vi "LBCB Cartesian Data.vi"() -> ()   [LabVIEW 2009]
uses:
  lib/Launcher/Launcher Actions.ctl
  lib/Launcher/NoPanelAppTypes.ctl
  lib/Data Access Objects/Metadata/DAO Actions.ctl
  lib/Data Access Objects/Application/Number Of LBCBs.ctl
  lib/Data Access Objects/Metadata/Persistant DAO Actions.ctl
panel:
  in  "Force Offset Tag":u16(ring)
  in  "Cartesian Type":bool caption="Coord"
  in  "Label1 3":string="Combined"
  in  "Label1 2":string="LBCB 2"
  in  "Label1":string="LBCB 1"
  out "Combined Data":dbl[][](array[numeric]) caption="LBCB 2 Data"
  out "DOF Labels3":string[](array[string])=["Dx", "Dy", "Dz", "Rx", "Ry", "Rz"]
  out "LBCB 1 Data":dbl[][](array[numeric])
  out "LBCB 2 Data":dbl[][](array[numeric])
  out "DOF Labels 2":string[](array[string])=["Dx", "Dy", "Dz", "Rx", "Ry", "Rz"]
  out "DOF Labels":string[](array[string])=["Dx", "Dy", "Dz", "Rx", "Ry", "Rz"]
  in  "Ok":bool
  # "Forces"
  # "Displacements"
  # "Commands"
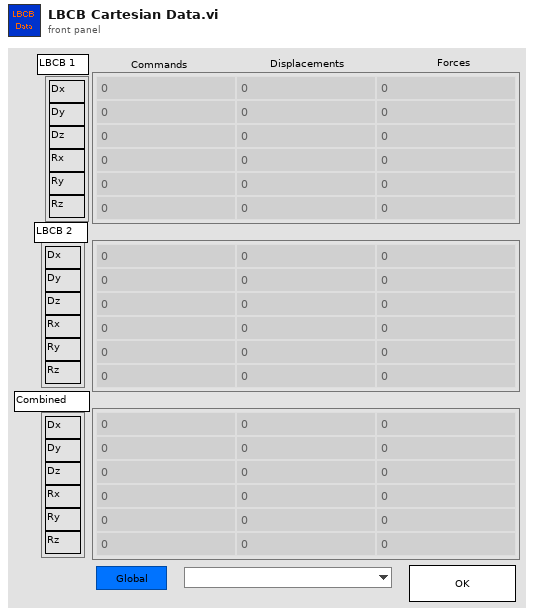
[diagram p1: front panel]
types:
  T1 = typedef "NoPanelAppTypes.ctl" = enum16{"NTCP Socket", "Data Archiving", "DAQ Link", "Control Loops", "Cmd Disp Diffs", "LBCB Cart Data", "Limits", "Mixed Mode Widget", "Offsets"}
  T2 = typedef "Launcher Actions.ctl" = enum16{"Launch", "Stop All", "Stop", "Kill", "Running?", "Init"}
  T3 = typedef "DAO Actions.ctl" = enum16{"Init", "Get", "Set"}
  T4 = typedef "Number Of LBCBs.ctl" = enum16{"1", "2"}
  T5 = typedef "Persistant DAO Actions.ctl" = enum16{"Init", "Get", "Set", "Load", "Save"}
  T6 = typedef "Dataset Source.ctl" = enum16{"LBCB 1", "LBCB 2", "Combined", "External Sensors"}
  T7 = typedef "Dataset Transaction Id.ctl" = cluster{"Dataset Source":T6, "Dataset Type":T8, "Hold":T9, "Volts":T9, "Tag":string}
  T8 = typedef "Dataset Type.ctl" = enum16{"LVDT", "Load Cell", "Actuator Command", "Servo Error", "Displacement Command", "Displacement", "Force"}
  T9 = typedef "Yes No Button.ctl" = bool
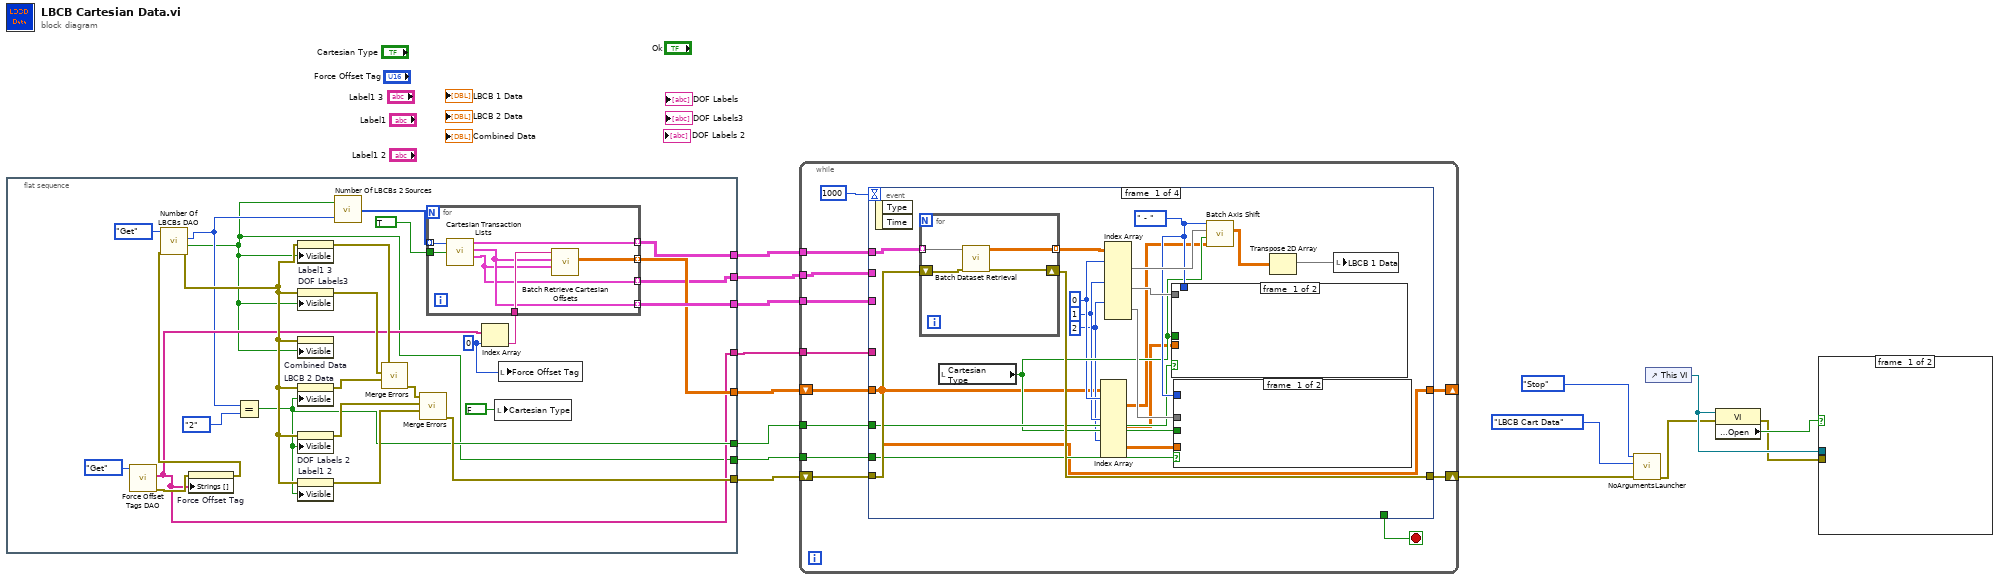
[diagram p0: block diagram]
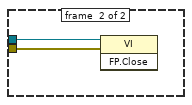
[diagram p2: hidden frame]
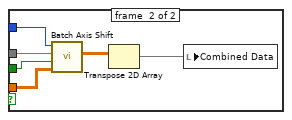
[diagram p3: hidden frame]
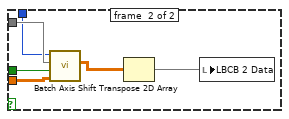
[diagram p4: hidden frame]
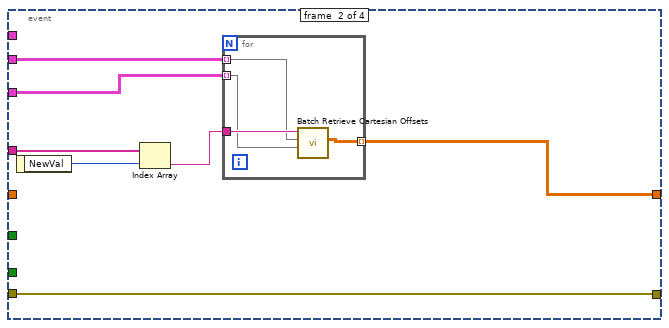
[diagram p5: hidden frame]
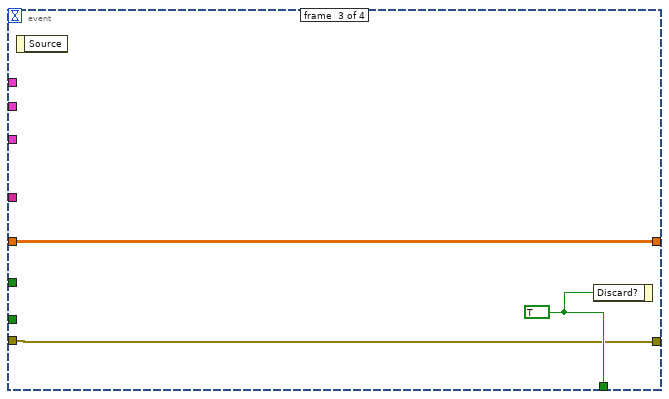
[diagram p6: hidden frame]
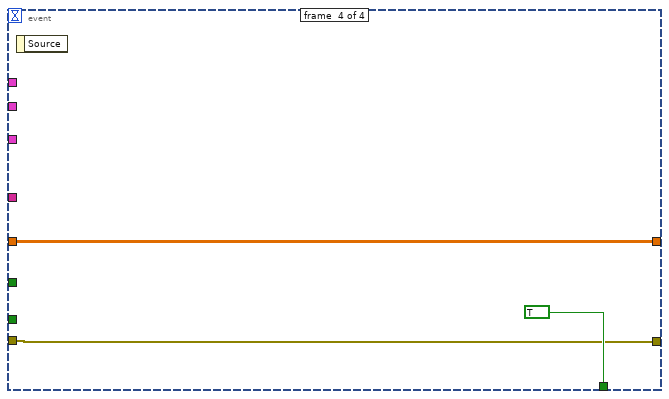
[diagram p7: hidden frame]
diagram:
  n1 = flat-sequence {
    tunnel: [w41] -> w12
    tunnel: [w25] -> w11
    tunnel: [w24] -> w10
    tunnel: [w18] -> w9
    tunnel: [w23] -> w8
    tunnel: [w22] -> w7
    tunnel: [w21] -> w6
    tunnel: [w20] -> w5
    frame #0 {
      w28 = 0 ("index")
      n2 = call "Force Offset Tags DAO.vi"("DAO Actions"=DAO_Actions."Get") -> ("error out"=w30:errorcluster, "Force Tags"=w20:string[])  [unwired: 9 in]
      n3 = property on="Force Offset Tag" class="Ring (strict)"(error in=w30, "Strings []"=w20) -> (error out=w29:errorcluster)  [unwired: 1 in, 1 out]
      n4 = call "Number Of LBCBs DAO.vi"("error in (no error)"=w29, "Actions"=Persistant_DAO_Actions."Get") -> ("error out"=w38:errorcluster, "Rigid Connection Out"=w18:bool, "Number of\nLBCBs Out"=w19:T4)  [unwired: 6 in, 1 out]
      n5 = Equal?(x=w19, y=Number_Of_LBCBs."2") -> (x = y?=w23:bool)
      n6 = property on="Label1 3" class="Str"(error in=w38, "Visible"=w18) -> (error out=w37:errorcluster)  [unwired: 1 in, 1 out]
      n7 = property on="DOF Labels3" class="Arr (strict)"(error in=w38, "Visible"=w18) -> (error out=w36:errorcluster)  [unwired: 1 in, 1 out]
      n8 = property on="Combined Data" class="Arr (strict)"(error in=w38, "Visible"=w18) -> ()  [unwired: 1 in, 2 out]
      n9 = property on="LBCB 2 Data" class="Arr (strict)"(error in=w38, "Visible"=w23) -> (error out=w35:errorcluster)  [unwired: 1 in, 1 out]
      n10 = property on="DOF Labels 2" class="Arr (strict)"(error in=w38, "Visible"=w23) -> (error out=w33:errorcluster)  [unwired: 1 in, 1 out]
      n11 = property on="Label1 2" class="Str"(error in=w38, "Visible"=w23) -> (error out=w32:errorcluster)  [unwired: 1 in, 1 out]
      n12 = call "Number Of LBCBs 2 Sources.vi"("Number of LBCBs"=w19, "Combined LBCBs"=w18) -> ("Sources"=w17:T6[])
      n13 = call <vilib>:"Merge Errors.vi"("error in 3 (no error)"=w35, "error in 2 (no error)"=w36, "error in 1 (no error)"=w37) -> ("error out"=w34:errorcluster)  [unwired: 4 in]
      n14 = call <vilib>:"Merge Errors.vi"("error in 3 (no error)"=w32, "error in 2 (no error)"=w33, "error in 1 (no error)"=w34) -> ("error out"=w41:errorcluster)  [unwired: 4 in]
      n15 = Index Array(array=w20, index=w28) -> (element=w26:string)
      n16 = for {
        tunnel: w26 -> [w48]
        tunnel: [w47] -> w25 mode=indexing
        tunnel: [w46] -> w24 mode=indexing
        tunnel: [w45] -> w22 mode=indexing
        tunnel: [w44] -> w21 mode=indexing
        tunnel: w17 -> [w43] mode=indexing
        tunnel: TRUE ("Include Command") -> [w42]
        n17 = call "Cartesian Transaction Lists.vi"("Source"=w43, "Include Command"=w42) -> ("Cartesian Data"=w47:T7[], "Displacement Offsets"=w46:T7[], "Force Offsets"=w44:T7[])  [unwired: 1 in, 1 out]
        n18 = call "Batch Retrieve Cartesian Offsets.vi"("Force Offsets"=w44, "Displacement Offsets"=w46, "Force Tag"=w48) -> ("Offsets"=w45:dbl[][])  [unwired: 5 in, 1 out]
      }
      n19 = local write "Cartesian Type"(FALSE ("Cartesian Type")) -> ()
      n20 = local write "Force Offset Tag"(w28) -> ()
    }
  }
  n21 = while {
    shift-right: [w57] -> w13
    shift-left: w12 -> [w58]
    tunnel: w11 -> [w56]
    tunnel: w10 -> [w50]
    tunnel: w9 -> [w55]
    tunnel: w8 -> [w54]
    shift-right: [w49] -> _
    shift-left: w7 -> [w53]
    tunnel: w6 -> [w51]
    tunnel: w5 -> [w52]
    stop <- w59 stop-if-true
    n22 = event shown="[3] Application Instance Close;  Panel Close" {
      selector: _ -> [_ _ _ _]
      dyn-events: _ -> [_ _ _ _]
      timeout: 1000 -> [_ _ _ _]
      tunnel: [_ _ w110 TRUE] -> w59
      tunnel: w58 -> [w80 w97 w109 w112]
      tunnel: [w79 w97 w109 w112] -> w57
      tunnel: w56 -> [w76 _ _ _]
      tunnel: w55 -> [w71 _ _ _]
      tunnel: w54 -> [w69 _ _ _]
      tunnel: w53 -> [w61 _ w108 w111]
      tunnel: w52 -> [_ w103 _ _]
      tunnel: w51 -> [_ w100 _ _]
      tunnel: w50 -> [_ w99 _ _]
      tunnel: [w61 w98 w108 w111] -> w49
      event #0 {
        w70 = enum16{" +", " - "}." - " ("Direction")
        w65 = 2 ("index (row)")
        w66 = 1 ("index (row)")
        w67 = 0 ("index (row)")
        n23 = event-data() -> ()  [unwired: 3 out]
        n24 = for {
          tunnel: w76 -> [w96] mode=indexing
          shift-right: [w94] -> w79
          shift-left: w80 -> [w95]
          tunnel: [w93] -> w78 mode=indexing
          n25 = call "Batch Dataset Retrieval.vi"("error in"=w95, "Transactions"=w96) -> ("error out"=w94:errorcluster, "Data"=w93:dbl[][])  [unwired: 8 in]
        }
        n26 = local read "Cartesian Type"() -> (w68:bool)
        n27 = Index Array(array=w61, index (dim 0) #1=w67, index (dim 0) #2=w66, index (dim 0) #3=w65) -> (element #1=w64:dbl[][], element #2=w63:dbl[][], element #3=w62:dbl[][])  [unwired: 6 in]
        n28 = Index Array(array=w78, index (dim 0) #1=w67, index (dim 0) #2=w66, index (dim 0) #3=w65) -> (element #1=w75:dbl[][], element #2=w73:dbl[][], element #3=w72:dbl[][])  [unwired: 6 in]
        n29 = case shown="True" w69 {
          tunnel: w73 -> [_ w91]
          tunnel: w70 -> [_ w89]
          tunnel: w68 -> [_ w88]
          tunnel: w63 -> [_ w87]
          frame #0 {
          }
          frame #1 {
            n30 = call "Batch Axis Shift.vi"("Offsets In"=w87, "Coordinate Switch"=w88, "Data In"=w91, "Direction"=w89) -> ("Data Out"=w90:dbl[][])  [unwired: 7 in]
            n31 = Transpose 2D Array(2D array=w90) -> (transposed array=w92:dbl[][])
            n32 = local write "LBCB 2 Data"(w92) -> ()
          }
        }
        n33 = case shown="True" w71 {
          tunnel: w72 -> [_ w85]
          tunnel: w70 -> [_ w83]
          tunnel: w68 -> [_ w82]
          tunnel: w62 -> [_ w81]
          frame #0 {
          }
          frame #1 {
            n34 = call "Batch Axis Shift.vi"("Offsets In"=w81, "Coordinate Switch"=w82, "Data In"=w85, "Direction"=w83) -> ("Data Out"=w84:dbl[][])  [unwired: 7 in]
            n35 = Transpose 2D Array(2D array=w84) -> (transposed array=w86:dbl[][])
            n36 = local write "Combined Data"(w86) -> ()
          }
        }
        n37 = call "Batch Axis Shift.vi"("Offsets In"=w64, "Coordinate Switch"=w68, "Data In"=w75, "Direction"=w70) -> ("Data Out"=w74:dbl[][])  [unwired: 7 in]
        n38 = Transpose 2D Array(2D array=w74) -> (transposed array=w77:dbl[][])
        n39 = local write "LBCB 1 Data"(w77) -> ()
      }
      event #1 {
        n40 = event-data() -> ("NewVal"=w102:u16)  [unwired: 1 out]
        n41 = Index Array(array=w103, index=w102) -> (element=w101:string)
        n42 = for {
          tunnel: w101 -> [w107]
          tunnel: w100 -> [w106] mode=indexing
          tunnel: w99 -> [w105] mode=indexing
          tunnel: [w104] -> w98 mode=indexing
          n43 = call "Batch Retrieve Cartesian Offsets.vi"("Force Offsets"=w105, "Displacement Offsets"=w106, "Force Tag"=w107) -> ("Offsets"=w104:dbl[][])  [unwired: 5 in, 1 out]
        }
      }
      event #2 {
        w110 = TRUE
        n44 = event-data() -> ()  [unwired: 2 out]
        n45 = event-data("Discard?"=w110) -> ()  [unwired: 1 in, 1 out]
      }
      event #3 {
        n46 = event-data() -> ()  [unwired: 2 out]
      }
    }
  }
  n47 = call "NoArgumentsLauncher.vi"("error in (no error)"=w13, "Application"=NoPanelAppTypes."LBCB Cart Data", "Application Launcher Actions"=Launcher_Actions."Stop") -> ("error out"=w2:errorcluster)  [unwired: 8 out]
  n48 = control-ref of="This VI"() -> (w4:refnum<vi>)
  n49 = property class="VI"(reference=w4, error in=w2) -> (error out=w1:errorcluster, "Front Panel.Open"=w3:bool)  [unwired: 1 out]
  n50 = case shown="True" w3 {
    tunnel: w1 -> [_ w115]
    tunnel: w4 -> [_ w114]
    frame #0 {
    }
    frame #1 {
      n51 = invoke class="VI" method="FP.Close"(reference=w114, error in=w115) -> ()  [unwired: 1 in, 3 out]
    }
  }
